vi "ChangeDeviceStatus.vi"() -> ()   [LabVIEW 2013]
panel:
  in  "Numeric":dbl
  # "A value > 0 initializes communication"
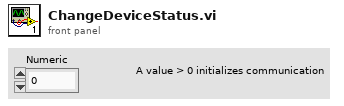
[diagram p1: front panel]
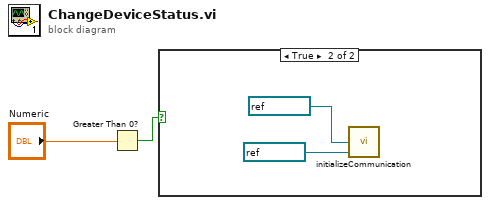
[diagram p0: block diagram]
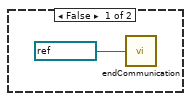
[diagram p2: hidden frame]
diagram:
  n1 = Greater Than 0?(x="Numeric") -> (x > 0?=w1:bool)
  n2 = case shown="True" w1 {
    frame False {
      n3 = call "endCommunication.vi"("Encoder COM Port"=refnum<visa-resource-name> "COM1" ("VRO COM Port")) -> ()  [unwired: 1 in]
    }
    frame True {
      n4 = call "initializeCommunication.vi"("Encoder COM Port"=refnum<visa-resource-name> "COM1" ("VROPort"), "Motor COM Port"=refnum<visa-resource-name> "COM4" ("VXM COM Port")) -> ()  [unwired: 1 in, 1 out]
    }
  }
